vi "ME_acquire.vi"() -> ()   [LabVIEW 2015]
doc: "Use this template to build a producer/consumer design pattern. Use this template when you need to execute a process, such as data analysis, when a data source, such as a triggered acquisition, produces data at an uneven rate and you need to execute the process when the data becomes available."
uses:
  oxford_driver/Oxford Drivers/BUSGEN.LLB/OxfordAddress.ctl
  <vilib>/Utility/file.llb/Write Delimited Spreadsheet (DBL).vi
  <vilib>/express/express arith-compare/Formula/XNode/ExpressFormulaBlockNode.xnode
panel:
  in  "Counter":dbl
  out "I(B) 3":cluster{dbl[], dbl[]}(graph)
  out "I(B) 2":cluster{dbl[], dbl[]}(graph)
  out "I(B)":cluster{dbl[], dbl[]}(graph)
  in  "Max Field (T)":dbl
  in  "Min Field (T)":dbl
  in  "Ramp up/down":bool
  out "I_T":cluster{dbl[], dbl[]}(graph)
  in  "Field To Zero":bool
  in  "Set Field (T)":dbl=0.3
  in  "Go to Set":bool
  out "L magnet (H)":dbl
  out "R magnet (mOhm)":dbl
  out "Actual Current (R0)":dbl
  out "Actual Field (T)":dbl
  out "Set":bool
  in  "Target Sweep Rate (T/min)":dbl=2.0 format="%.6f"
  out "Temperature array":dbl[](array[numeric])
  in  "New Measurement File":bool
  out "Measurement File":path
  out "refnum out":refnum<file>
  in  "Sampling rate (Hz)":dbl=20.0
  in  "Measuring":bool
  out "Actual Temperature (K)":dbl
  in  "Temp Refresh (s)":dbl=1.0
  in  "Lake Shore":refnum<visa-resource-name>="GPIB0::11::INSTR"
  out "Time Lag":dbl=0.0500025749206543
  out "Magnetic Field":cluster{dbl[], dbl[]}(graph)
  out "IV converter":cluster{dbl[], dbl[]}(graph)
  in  "Measure (Start/Pause)":bool
  in  "Magnetic Field":refnum<visa-resource-name>="GPIB0::21::INSTR"
  in  "IV converter":refnum<visa-resource-name>="GPIB0::20::INSTR"
  in  "stop":bool
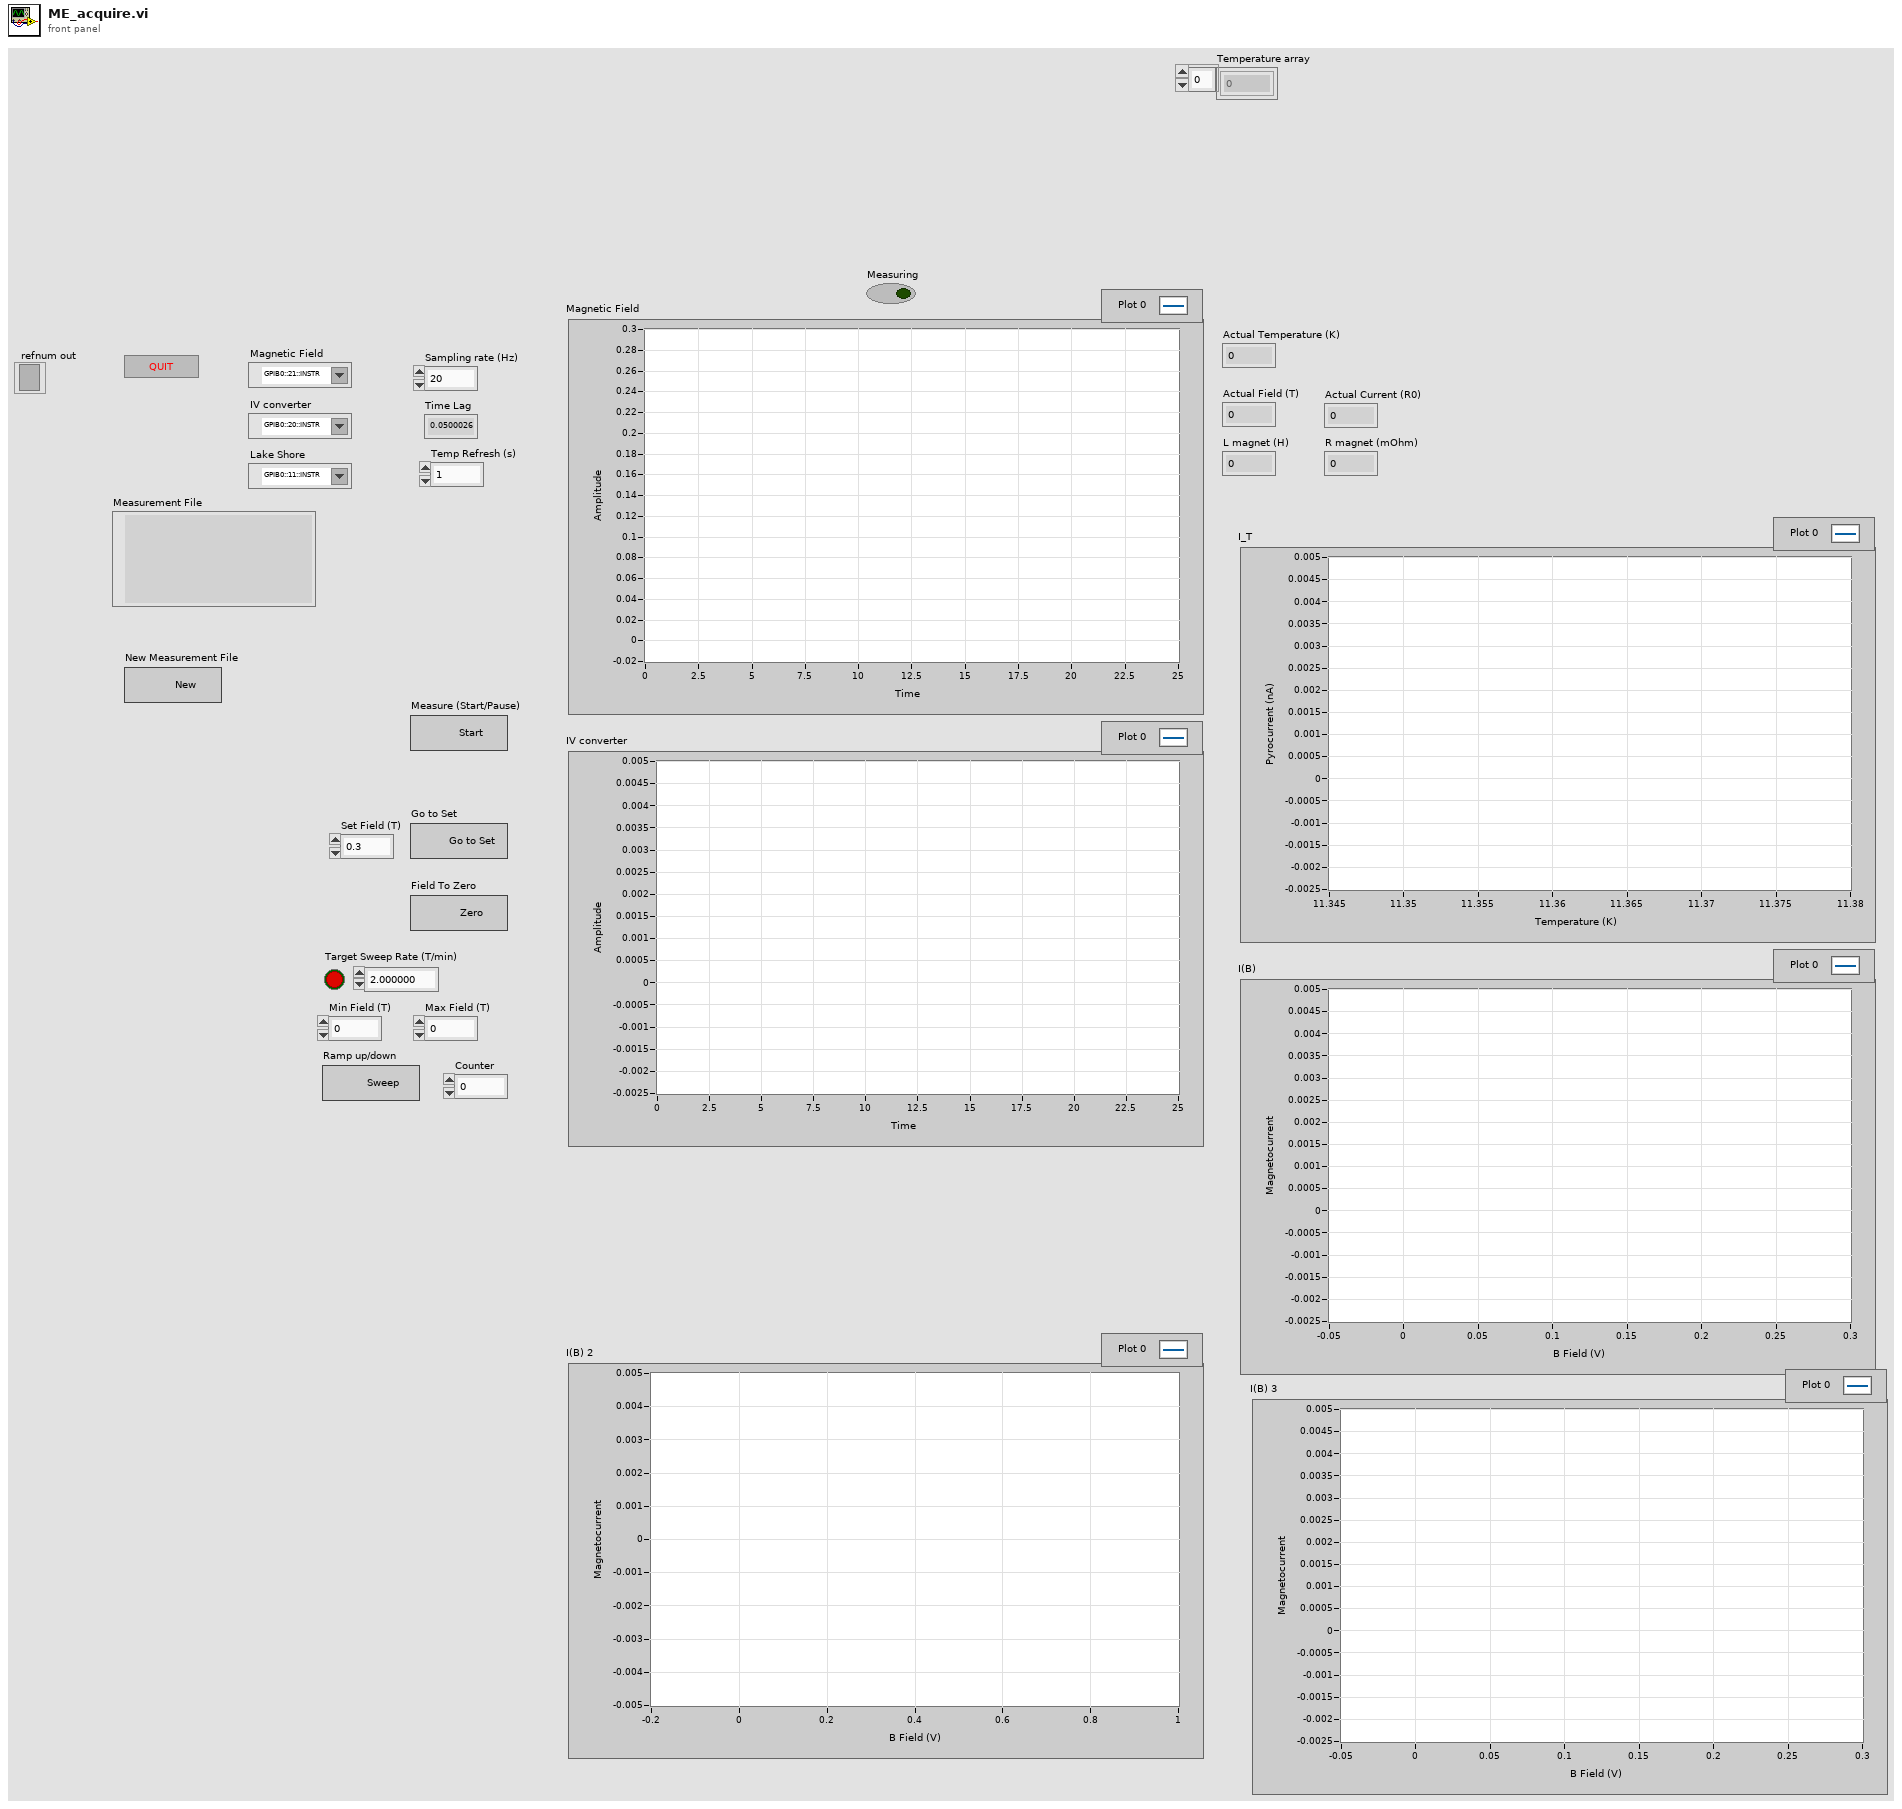
[diagram p1: front panel]
types:
  T1 = enum16{"open", "replace", "create", "open or create", "replace or create", "replace or create with confirmation"}
  T2 = typedef "OxfordAddress.ctl" = cluster{"Com Port":i32, "ISOBUS Address":i32, "GPIB Address":i16, "Communication":enum16{"RS232", "ISOBUS", "GPIB", "Gateway"}}
  T3 = cluster{"seconds since 1Jan1904":timestamp, "read buffer":string, "read buffer":string}
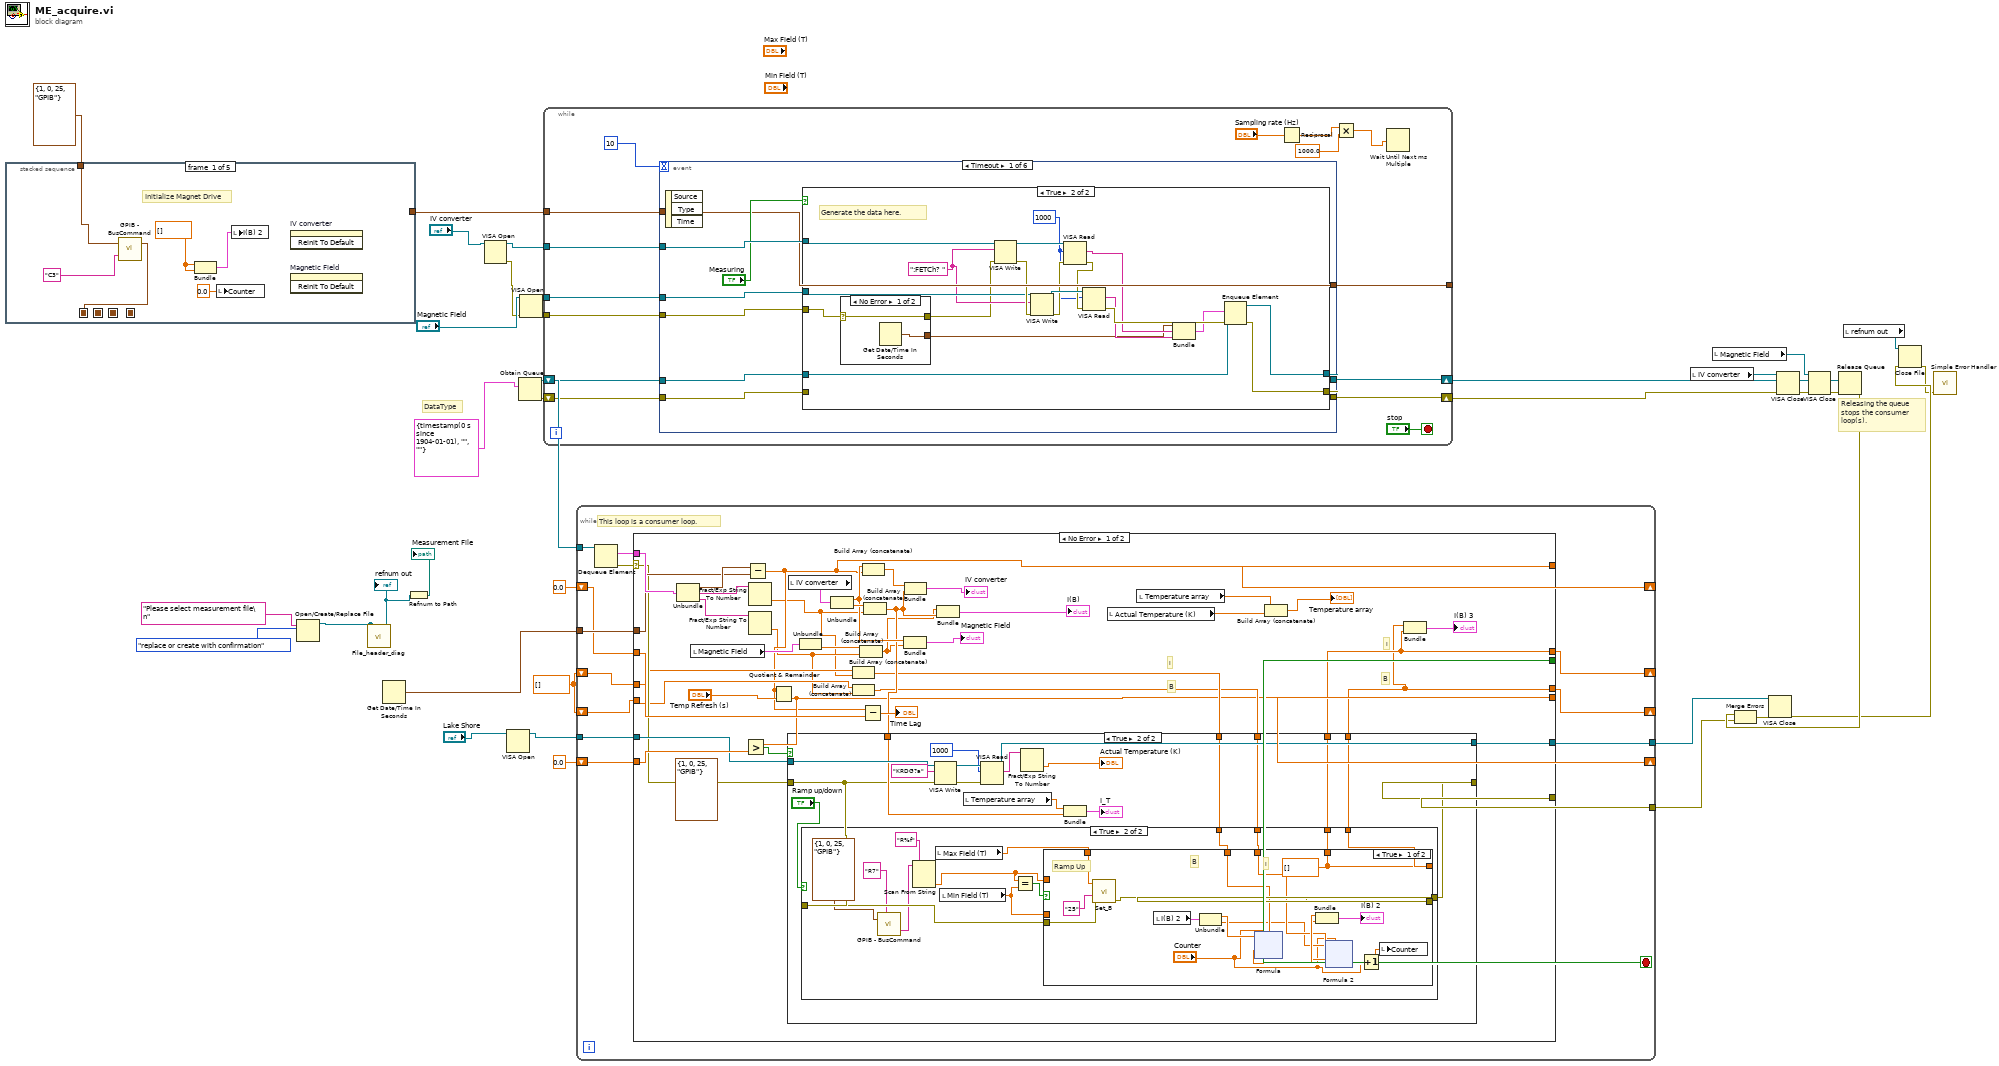
[diagram p0: block diagram]
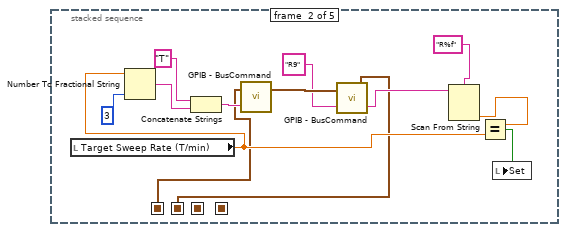
[diagram p2: hidden frame]
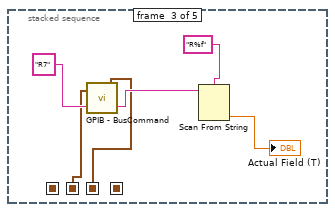
[diagram p3: hidden frame]
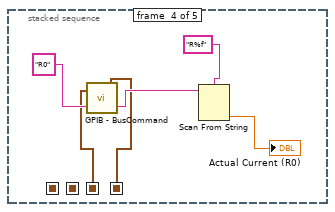
[diagram p4: hidden frame]
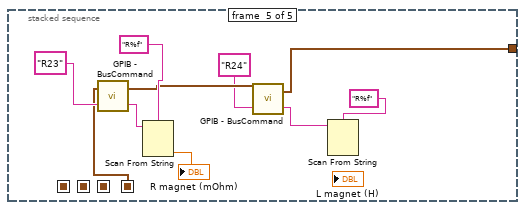
[diagram p5: hidden frame]
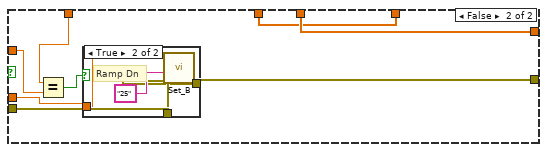
[diagram p8: hidden frame]
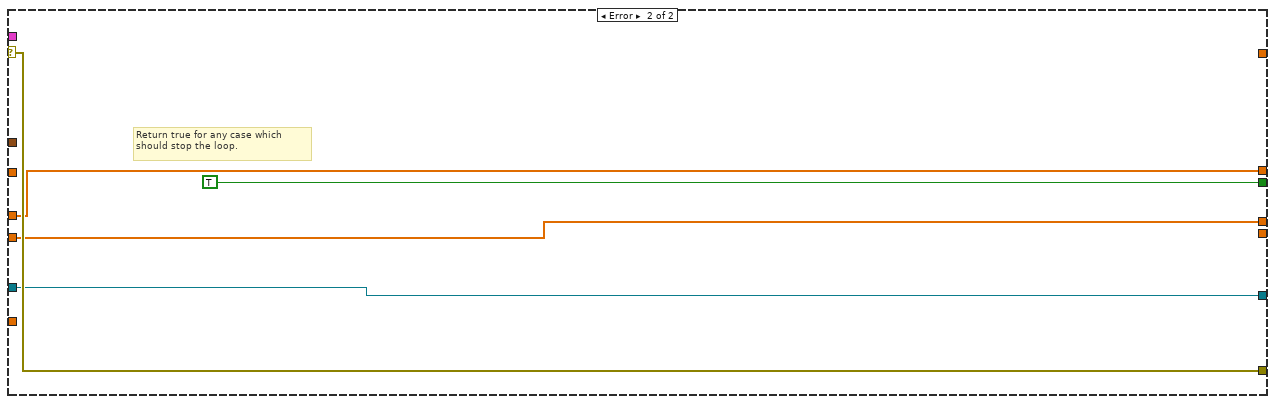
[diagram p10: hidden frame]
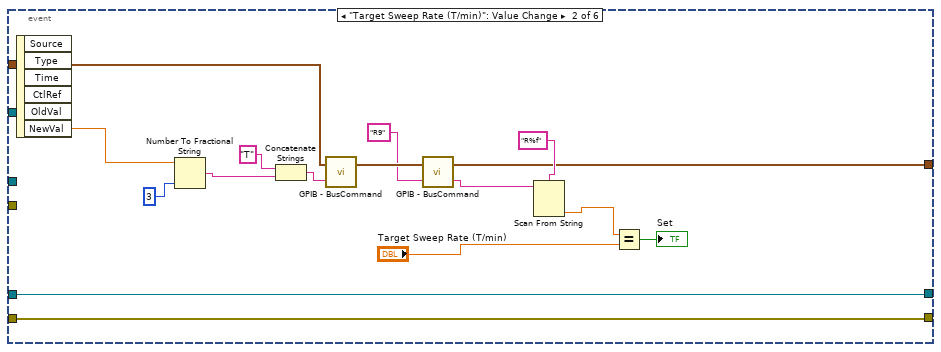
[diagram p13: hidden frame]
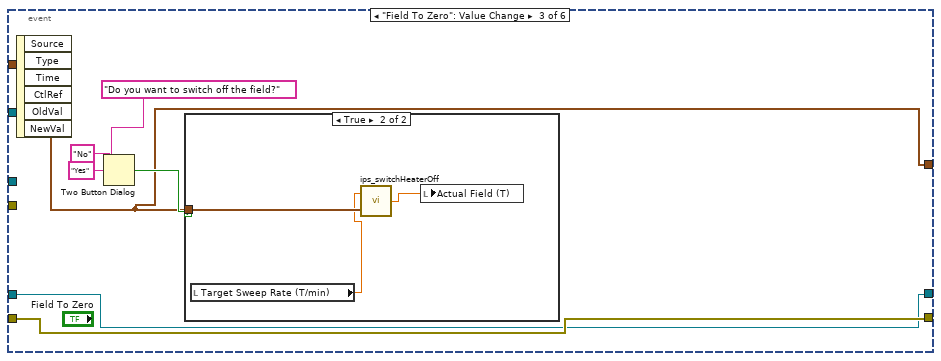
[diagram p14: hidden frame]
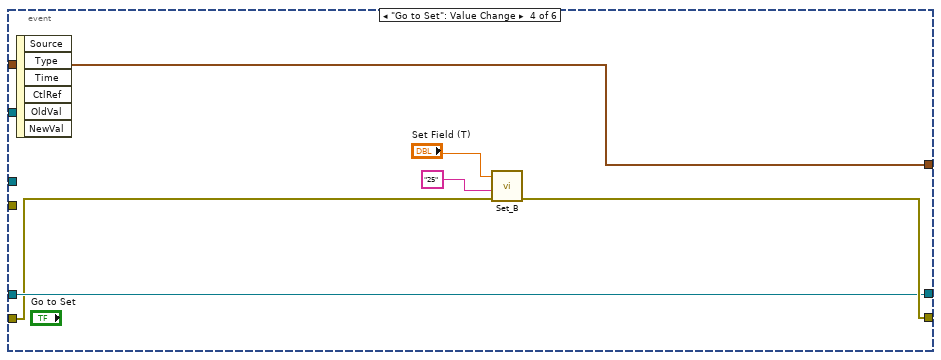
[diagram p16: hidden frame]
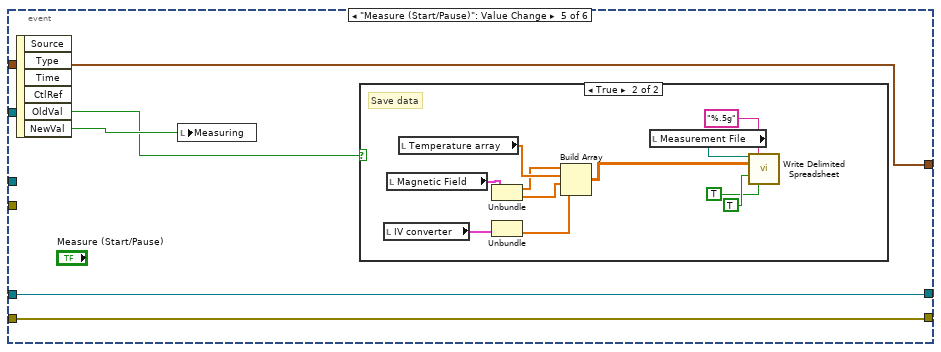
[diagram p17: hidden frame]
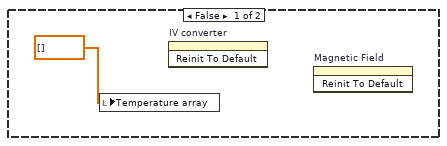
[diagram p18: hidden frame]
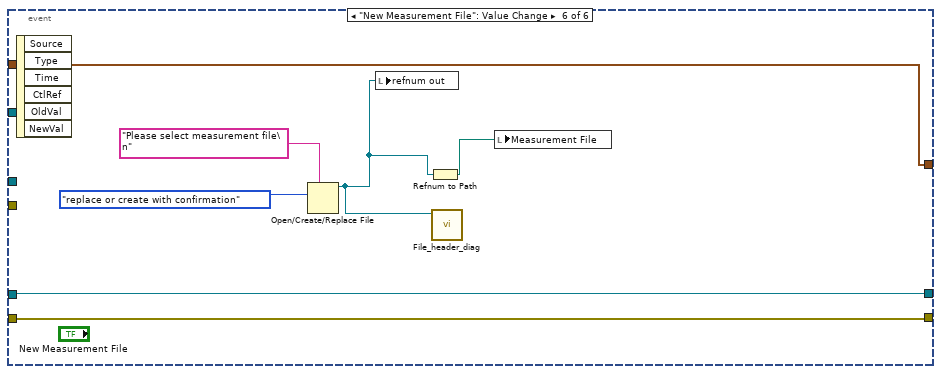
[diagram p19: hidden frame]
diagram:
  w5 = dbl[] []
  # "DataType"
  # "Releasing the queue stops the consumer loop(s)."
  n1 = stacked-sequence {
    seq-local: [w38 _ _ _ _] -> [_ w42 _ _ _]
    seq-local: [_ w41 _ _ _] -> [_ _ w55 _ _]
    seq-local: [_ _ w54 _ _] -> [_ _ _ w61 _]
    seq-local: [_ _ _ w60 _] -> [_ _ _ _ w71]
    tunnel: T2 {"Com Port"=1, "ISOBUS Address"=0, "GPIB Address"=25, "Communication"=enum."GPIB"} ("Address") -> [w39 _ _ _ _]
    tunnel: [_ _ _ _ w69] -> w6
    frame #0 {
      w35 = dbl[] [] ("Result")
      # "Initialize Magnet Drive"
      n2 = call "GPIB - BusCommand.vi"("Command"="C3", "Address"=w39) -> ("Address(thru)"=w38:T2)  [unwired: 1 out]
      n3 = Bundle("Result"=w35, "Result"=w35) -> (w36:cluster{"Result":dbl[], "Result":dbl[]})  [unwired: 1 in]
      n4 = local write "Counter"(0.0 ("Counter")) -> ()
      n5 = local write "I(B) 2"(w36) -> ()
      n6 = invoke on="IV converter" class="XYGraph (strict)" method="Reinit To Default"() -> ()  [unwired: 3 in, 3 out]
      n7 = invoke on="Magnetic Field" class="XYGraph (strict)" method="Reinit To Default"() -> ()  [unwired: 3 in, 3 out]
    }
    frame #1 {
      n8 = local read "Target Sweep Rate (T/min)"() -> (w44:dbl)
      n9 = Number To Fractional String(number=w44, precision (6)=i16 3) -> (F-format string=w51:string)  [unwired: 2 in]
      n10 = Concatenate Strings("T" ("format string"), w51) -> (w50:string)
      n11 = call "GPIB - BusCommand.vi"("Command"=w50, "Address"=w42) -> ("Address(thru)"=w49:T2)  [unwired: 1 out]
      n12 = call "GPIB - BusCommand.vi"("Command"="R9" ("format string"), "Address"=w49) -> ("Reply"=w47:string, "Address(thru)"=w41:T2)
      n13 = Scan From String(format string="R%f" ("remaining string"), input string=w47) -> (output 1=w45:dbl)  [unwired: 3 in, 3 out]
      n14 = Equal?(x=w45, y=w44) -> (x = y?=w43:bool)
      n15 = local write "Set"(w43) -> ()
    }
    frame #2 {
      n16 = call "GPIB - BusCommand.vi"("Command"="R7" ("format string"), "Address"=w55) -> ("Reply"=w59:string, "Address(thru)"=w54:T2)
      n17 = Scan From String(format string="R%f" ("remaining string"), input string=w59) -> (output 1=→"Actual Field (T)":dbl)  [unwired: 3 in, 3 out]
    }
    frame #3 {
      n18 = call "GPIB - BusCommand.vi"("Command"="R0" ("format string"), "Address"=w61) -> ("Reply"=w65:string, "Address(thru)"=w60:T2)
      n19 = Scan From String(format string="R%f" ("remaining string"), input string=w65) -> (output 1=→"Actual Current (R0)":dbl)  [unwired: 3 in, 3 out]
    }
    frame #4 {
      n20 = call "GPIB - BusCommand.vi"("Command"="R23" ("format string"), "Address"=w71) -> ("Reply"=w75:string, "Address(thru)"=w70:T2)
      n21 = Scan From String(format string="R%f" ("remaining string"), input string=w75) -> (output 1=→"R magnet (mOhm)":dbl)  [unwired: 3 in, 3 out]
      n22 = call "GPIB - BusCommand.vi"("Command"="R24" ("format string"), "Address"=w70) -> ("Reply"=w67:string, "Address(thru)"=w69:T2)
      n23 = Scan From String(format string="R%f" ("remaining string"), input string=w67) -> ()  [unwired: 4 in, 3 out]
    }
  }
  n24 = Open/Create/Replace File(prompt="Please select measurement file\n", operation (0:open)=T1."replace or create with confirmation") -> (refnum out=w1:refnum<file>)  [unwired: 4 in, 2 out]
  "refnum out" <- w1
  n25 = call "File_header_diag.vi"("Byte Stream File in"=w1) -> ()  [unwired: 11 in]
  n26 = Get Date/Time In Seconds() -> (seconds since 1Jan1904=w19:timestamp)
  n27 = Refnum to Path(1:w1) -> (0:→"Measurement File":path)
  n28 = VISA Open(VISA resource name="IV converter") -> (VISA resource name=w28:refnum<visa-resource-name>, error out=w30:errorcluster)  [unwired: 4 in]
  n29 = VISA Open(VISA resource name="Lake Shore") -> (VISA resource name=w17:refnum<visa-resource-name>)  [unwired: 4 in, 1 out]
  n30 = Obtain Queue(element data type=T3 {"seconds since 1Jan1904"=timestamp(0 s since 1904-01-01), "read buffer"="", "read buffer"=""} ("output cluster")) -> (queue out=w34:refnum<queue>, error out=w33:errorcluster)  [unwired: 4 in, 1 out]
  n31 = VISA Open(error in (no error)=w30, VISA resource name="Magnetic Field") -> (VISA resource name=w27:refnum<visa-resource-name>, error out=w26:errorcluster)  [unwired: 3 in]
  n32 = while {
    shift-right: [w86] -> w24
    shift-left: w33 -> [w87]
    shift-right: [w88] -> w32
    shift-left: w34 -> [w89]
    tunnel: w28 -> [w85]
    tunnel: w27 -> [w84]
    tunnel: w26 -> [w83]
    tunnel: [w77] -> _
    tunnel: w6 -> [w76]
    stop <- "stop" stop-if-true
    n33 = event shown="[0] Timeout" {
      selector: _ -> [_ _ _ _ _ _]
      dyn-events: _ -> [_ _ _ _ _ _]
      timeout: 10 -> [_ _ _ _ _ _]
      tunnel: w89 -> [w99 w125 w141 w152 w160 w174]
      tunnel: [w98 w125 w141 w152 w160 w174] -> w88
      tunnel: w87 -> [w97 w124 w142 w151 w159 w175]
      tunnel: [w96 w124 w142 w153 w159 w175] -> w86
      tunnel: w85 -> [w95 _ _ _ _ _]
      tunnel: w84 -> [w94 _ _ _ _ _]
      tunnel: w83 -> [w93 _ _ _ _ _]
      tunnel: [w91 w130 w140 w154 w156 w173] -> w77
      tunnel: w76 -> [w91 w126 w140 w154 w156 w173]
      event Timeout {
        n34 = event-data() -> ()  [unwired: 1 in, 3 out]
        n35 = case shown="True" "Measuring" {
          tunnel: w99 -> [w101 w120]
          tunnel: [w101 w119] -> w98
          tunnel: w97 -> [w100 _]
          tunnel: [w100 w118] -> w96
          tunnel: w95 -> [_ w111]
          tunnel: w94 -> [_ w110]
          tunnel: w93 -> [_ w105]
          frame False {
          }
          frame True {
            w108 = ":FETCh? " ("data")
            w112 = u32 1000 ("byte count")
            # "Generate the data here."
            n36 = case shown="No Error" w105 {
              selector: w105 -> [w122 w123]
              tunnel: [w122 w123] -> w104
              tunnel: [w121 _] -> w103
              frame No Error {
                n37 = Get Date/Time In Seconds() -> (seconds since 1Jan1904=w121:timestamp)
              }
              frame Error {
              }
            }
            n38 = VISA Write(VISA resource name=w111, write buffer=w108, error in (no error)=w104) -> (VISA resource name out=w117:refnum<visa-resource-name>, error out=w115:errorcluster)  [unwired: 1 out]
            n39 = VISA Write(VISA resource name=w110, write buffer=w108, error in (no error)=w115) -> (VISA resource name out=w116:refnum<visa-resource-name>, error out=w114:errorcluster)  [unwired: 1 out]
            n40 = VISA Read(VISA resource name=w117, byte count=w112, error in (no error)=w114) -> (read buffer=w106:string, error out=w113:errorcluster)  [unwired: 2 out]
            n41 = VISA Read(VISA resource name=w116, byte count=w112, error in (no error)=w113) -> (read buffer=w107:string, error out=w109:errorcluster)  [unwired: 2 out]
            n42 = Bundle("seconds since 1Jan1904"=w103, "read buffer"=w106, "read buffer"=w107) -> (w102:T3)  [unwired: 1 in]
            n43 = Enqueue Element(queue=w120, element=w102, error in (no error)=w109) -> (queue out=w119:refnum<queue>, error out=w118:errorcluster)  [unwired: 1 in, 1 out]
          }
        }
      }
      event "Target Sweep Rate (T/min)": Value Change {
        n44 = event-data() -> ("NewVal"=w138:dbl)  [unwired: 1 in, 5 out]
        n45 = Number To Fractional String(number=w138, precision (6)=i16 3) -> (F-format string=w136:string)  [unwired: 2 in]
        n46 = Concatenate Strings("T" ("format string"), w136) -> (w135:string)
        n47 = call "GPIB - BusCommand.vi"("Command"=w135, "Address"=w126) -> ("Address(thru)"=w134:T2)  [unwired: 1 out]
        n48 = call "GPIB - BusCommand.vi"("Command"="R9" ("format string"), "Address"=w134) -> ("Reply"=w132:string, "Address(thru)"=w130:T2)
        n49 = Scan From String(format string="R%f" ("remaining string"), input string=w132) -> (output 1=w129:dbl)  [unwired: 3 in, 3 out]
        n50 = Equal?(x=w129, y="Target Sweep Rate (T/min)") -> (x = y?=→"Set":bool)
      }
      event "Field To Zero": Value Change {
        n51 = event-data() -> ()  [unwired: 1 in, 6 out]
        n52 = Two Button Dialog(message="Do you want to switch off the field?", 1:"No" ("F button name (\"Cancel\")"), 2:"Yes" ("T button name (\"OK\")")) -> (T button?=w146:bool)
        n53 = case shown="True" w146 {
          tunnel: w140 -> [_ w149]
          frame False {
          }
          frame True {
            n54 = local read "Target Sweep Rate (T/min)"() -> (w148:dbl)
            n55 = call "ips_switchHeaterOff.vi"("Instrument address"=w149, "Rate"=w148) -> ("B"=w147:dbl)
            n56 = local write "Actual Field (T)"(w147) -> ()
          }
        }
      }
      event "Go to Set": Value Change {
        n57 = event-data() -> ()  [unwired: 1 in, 6 out]
        n58 = call "Set_B.vi"("error in (no error)"=w151, "address string"="25", "Set Field (T)"="Set Field (T)") -> ("error out"=w153:errorcluster)  [unwired: 8 in]
      }
      event "Measure (Start/Pause)": Value Change {
        n59 = event-data() -> ("OldVal"=w157:bool, "NewVal"=w158:bool)  [unwired: 1 in, 4 out]
        n60 = local write "Measuring"(w158) -> ()
        n61 = case shown="True" w157 {
          frame False {
            n62 = local write "Temperature array"(dbl[] []) -> ()
            n63 = invoke on="IV converter" class="XYGraph (strict)" method="Reinit To Default"() -> ()  [unwired: 3 in, 3 out]
            n64 = invoke on="Magnetic Field" class="XYGraph (strict)" method="Reinit To Default"() -> ()  [unwired: 3 in, 3 out]
          }
          frame True {
            # "Save data"
            n65 = local read "IV converter"() -> (w167:cluster{dbl[], dbl[]})
            n66 = local read "Magnetic Field"() -> (w166:cluster{dbl[], dbl[]})
            n67 = local read "Temperature array"() -> (w172:dbl[])
            n68 = Unbundle(w166) -> (w165:dbl[], w164:dbl[])
            n69 = Unbundle(w167) -> (w163:dbl[])  [unwired: 1 out]
            n70 = Build Array(w165, w172, w164, w163) -> (w169:dbl[][])
            n71 = local read "Measurement File"() -> (w170:path)
            n72 = call-poly <vilib>:"Write Delimited Spreadsheet.vi"("file path (dialog if empty)"=w170, "format (%.3f)"="%.5g", "2D data"=w169, "append to file? (F)"=TRUE, "transpose? (F)"=TRUE) -> ()  [unwired: 9 in, 2 out]
          }
        }
      }
      event "New Measurement File": Value Change {
        n73 = event-data() -> ()  [unwired: 1 in, 6 out]
        n74 = Open/Create/Replace File(prompt="Please select measurement file\n", operation (0:open)=T1."replace or create with confirmation") -> (refnum out=w176:refnum<file>)  [unwired: 4 in, 2 out]
        n75 = local write "refnum out"(w176) -> ()
        n76 = Refnum to Path(1:w176) -> (0:w177:path)
        n77 = call "File_header_diag.vi"("Byte Stream File in"=w176) -> ()  [unwired: 11 in]
        n78 = local write "Measurement File"(w177) -> ()
      }
    }
    n79 = Reciprocal(x="Sampling rate (Hz)") -> (1/x=w81:dbl)
    n80 = Multiply(x=w81, y=1000.0) -> (x*y=w79:dbl)
    n81 = Wait Until Next ms Multiple(millisecond multiple=w79) -> ()  [unwired: 1 out]
  }
  n82 = while {
    tunnel: w34 -> [w195]
    tunnel: w19 -> [w191]
    shift-right: [w190] -> _
    shift-left: 0.0 -> [w189]
    tunnel: w17 -> [w188]
    shift-right: [w187] -> _
    shift-left: 0.0 -> [w186]
    tunnel: [w185] -> w11
    tunnel: [w184] -> w14
    shift-right: [w180] -> _
    shift-left: w5 -> [w183]
    shift-right: [w181] -> _
    shift-left: w5 -> [w182]
    stop <- w192 stop-if-true
    # "This loop is a consumer loop."
    n83 = Dequeue Element(queue=w195) -> (element=w193:T3, error out=w194:errorcluster)  [unwired: 2 in, 2 out]
    n84 = case shown="No Error" w194 {
      selector: w194 -> [w221 w337]
      tunnel: w193 -> [w234 _]
      tunnel: [_ TRUE] -> w192
      tunnel: w191 -> [w230 _]
      tunnel: [w199 _] -> w190
      tunnel: w189 -> [w227 _]
      tunnel: w188 -> [w222 w336]
      tunnel: [w202 _] -> w187
      tunnel: w186 -> [w224 _]
      tunnel: [w220 w337] -> w185
      tunnel: [w219 w336] -> w184
      tunnel: [w201 w334] -> w180
      tunnel: w183 -> [w206 w334]
      tunnel: w182 -> [w204 w335]
      tunnel: [w200 w335] -> w181
      frame No Error {
        (unwired) T2 {"Com Port"=1, "ISOBUS Address"=0, "GPIB Address"=25, "Communication"=enum."GPIB"} ("Address")
        # "B"
        # "I"
        # "I"
        # "B"
        n85 = Unbundle(w234) -> ("seconds since 1Jan1904"=w231:timestamp, "read buffer"=w233:string, "read buffer"=w232:string)
        n86 = local read "Magnetic Field"() -> (w215:cluster{dbl[], dbl[]})
        n87 = Subtract(x=w231, y=w230) -> (x-y=w199:dbl)
        n88 = Fract/Exp String To Number(string=w233) -> (number=w196:dbl)  [unwired: 3 in, 1 out]
        n89 = Fract/Exp String To Number(string=w232) -> (number=w198:dbl)  [unwired: 3 in, 1 out]
        n90 = Quotient & Remainder(x=w199, y="Temp Refresh (s)") -> (floor(x/y)=w202:dbl)  [unwired: 1 out]
        n91 = Greater?(x=w202, y=w224) -> (0:w223:bool)
        n92 = local read "IV converter"() -> (w213:cluster{dbl[], dbl[]})
        n93 = Unbundle(w215) -> (w214:dbl[])  [unwired: 1 out]
        n94 = Unbundle(w213) -> (w210:dbl[], w212:dbl[])
        n95 = Build Array (concatenate)(w206, w196) -> (w205:dbl[])
        n96 = Build Array (concatenate)(w204, w198) -> (w203:dbl[])
        n97 = Build Array (concatenate)(w214, w198) -> (w207:dbl[])
        n98 = Subtract(x=w199, y=w227) -> (x-y=→"Time Lag":dbl)
        n99 = Build Array (concatenate)(w210, w199) -> (w211:dbl[])
        n100 = Build Array (concatenate)(w212, w196) -> (w209:dbl[])
        n101 = case shown="True" w223 {
          tunnel: w222 -> [w237 w256]
          tunnel: w221 -> [w238 w245]
          tunnel: [w238 w244] -> w220
          tunnel: [w237 w250] -> w219
          tunnel: w209 -> [_ w247]
          tunnel: w205 -> [w235 w242]
          tunnel: w203 -> [w236 w241]
          tunnel: [w235 w240] -> w201
          tunnel: [w236 w239] -> w200
          frame False {
          }
          frame True {
            n102 = case shown="True" "Ramp up/down" {
              tunnel: w245 -> [w259 w273]
              tunnel: [w259 w272] -> w244
              tunnel: w242 -> [w257 w263]
              tunnel: w241 -> [w258 w262]
              tunnel: [w257 w261] -> w240
              tunnel: [w258 w260] -> w239
              frame False {
              }
              frame True {
                n103 = call "GPIB - BusCommand.vi"("Command"="R7" ("format string"), "Address"=T2 {"Com Port"=1, "ISOBUS Address"=0, "GPIB Address"=25, "Communication"=enum."GPIB"}) -> ("Reply"=w268:string)  [unwired: 1 out]
                n104 = Scan From String(format string="R%f" ("remaining string"), input string=w268) -> (output 1=w265:dbl)  [unwired: 3 in, 3 out]
                n105 = local read "Max Field (T)"() -> (w270:dbl)
                n106 = local read "Min Field (T)"() -> (w269:dbl)
                n107 = Equal?(x=w265, y=w269) -> (x = y?=w271:bool)
                n108 = case shown="True" w271 {
                  tunnel: w273 -> [w287 w328]
                  tunnel: [w283 w327] -> w272
                  tunnel: w270 -> [w286 w325]
                  tunnel: w265 -> [_ w326]
                  tunnel: w269 -> [_ w324]
                  tunnel: w263 -> [w280 w321]
                  tunnel: w262 -> [w278 w322]
                  tunnel: [w284 w321] -> w261
                  tunnel: [w284 w322] -> w260
                  frame True {
                    w284 = dbl[] []
                    # "I"
                    # "B"
                    # "Ramp Up"
                    n109 = call "Set_B.vi"("error in (no error)"=w287, "address string"="25", "Set Field (T)"=w286) -> ("error out"=w283:errorcluster)  [unwired: 8 in]
                    n110 = local read "I(B) 2"() -> (w285:cluster{dbl[], dbl[]})
                    n111 = Unbundle(w285) -> (w281:dbl[], w277:dbl[])
                    n112 = xnode "Formula"("X"=w281, "count"="Counter", "Xnew"=w280) -> ("Result"=w279:dbl[])  [unwired: 1 in, 1 out]
                    n113 = xnode "Formula 2"("X"=w277, "count"="Counter", "Xnew"=w278) -> ("Result"=w276:dbl[])  [unwired: 1 in, 1 out]
                    n114 = Bundle("Result"=w279, "Result"=w276) -> (→"I(B) 2":cluster{"Result":dbl[], "Result":dbl[]})  [unwired: 1 in]
                    n115 = Increment(x="Counter") -> (x+1=w274:dbl)
                    n116 = local write "Counter"(w274) -> ()
                  }
                  frame False {
                    n117 = Equal?(x=w325, y=w326) -> (x = y?=w323:bool)
                    n118 = case shown="True" w323 {
                      tunnel: w328 -> [w329 w332]
                      tunnel: [w329 w331] -> w327
                      tunnel: w324 -> [_ w330]
                      frame False {
                      }
                      frame True {
                        # "Ramp Dn"
                        n119 = call "Set_B.vi"("error in (no error)"=w332, "address string"="25", "Set Field (T)"=w330) -> ("error out"=w331:errorcluster)  [unwired: 8 in]
                      }
                    }
                  }
                }
              }
            }
            n120 = VISA Write(VISA resource name=w256, write buffer="KRDG?a", error in (no error)=w245) -> (VISA resource name out=w254:refnum<visa-resource-name>, error out=w253:errorcluster)  [unwired: 1 out]
            n121 = local read "Temperature array"() -> (w248:dbl[])
            n122 = VISA Read(VISA resource name=w254, byte count=u32 1000, error in (no error)=w253) -> (VISA resource name out=w250:refnum<visa-resource-name>, read buffer=w251:string)  [unwired: 2 out]
            n123 = Fract/Exp String To Number(string=w251) -> (number=→"Actual Temperature (K)":dbl)  [unwired: 3 in, 1 out]
            n124 = Bundle("Temperature array"=w248, w247) -> (→"I_T":cluster{"Temperature array":dbl[], dbl[]})  [unwired: 1 in]
          }
        }
        n125 = Bundle(w210, w207) -> (→"Magnetic Field":cluster{dbl[], dbl[]})  [unwired: 1 in]
        n126 = Bundle(w211, w209) -> (→"IV converter":cluster{dbl[], dbl[]})  [unwired: 1 in]
        n127 = Bundle(w207, w209) -> (→"I(B)":cluster{dbl[], dbl[]})  [unwired: 1 in]
        n128 = local read "Actual Temperature (K)"() -> (w218:dbl)
        n129 = local read "Temperature array"() -> (w216:dbl[])
        n130 = Build Array (concatenate)(w216, w218) -> (→"Temperature array":dbl[])
        n131 = Bundle(w200, w201) -> (→"I(B) 3":cluster{dbl[], dbl[]})  [unwired: 1 in]
      }
      frame Error {
        # "Return true for any case which should stop the loop."
      }
    }
  }
  n132 = local read "IV converter"() -> (w22:refnum<visa-resource-name>)
  n133 = local read "Magnetic Field"() -> (w21:refnum<visa-resource-name>)
  n134 = VISA Close(VISA resource name=w22, error in (no error)=w24) -> (error out=w25:errorcluster)
  n135 = VISA Close(VISA resource name=w21, error in (no error)=w25) -> (error out=w23:errorcluster)
  n136 = Release Queue(queue=w32, error in (no error)=w23) -> (error out=w12:errorcluster)  [unwired: 1 in, 2 out]
  n137 = Merge Errors(w12, w11) -> (w13:errorcluster)
  n138 = VISA Close(VISA resource name=w14, error in (no error)=w13) -> (error out=w10:errorcluster)
  n139 = local read "refnum out"() -> (w8:refnum<file>)
  n140 = Close File(refnum=w8, error in=w10) -> (error out=w9:errorcluster)  [unwired: 1 out]
  n141 = call <vilib>:"Simple Error Handler.vi"("error in (no error)"=w9) -> ()  [unwired: 4 in, 5 out]
